vi "Launch Worker Loop.vi"(8 "error in (no error)":errorcluster, 11 "ErrorFormat":refnum<class "IErrorFormat.lvclass">) -> (0 "error out":errorcluster, 3 "Queue Reference":refnum<data-value>)   [LabVIEW 2018, in "MVA Framework.lvlib" / "Composed Log.lvlib" / "Application Logger.lvclass"]
uses:
  Application Logger.lvclass
  Worker Loop.vi
  Types/MessageCluster.ctl
  Composed Log.lvlib
  IErrorFormat/IErrorFormat.lvclass
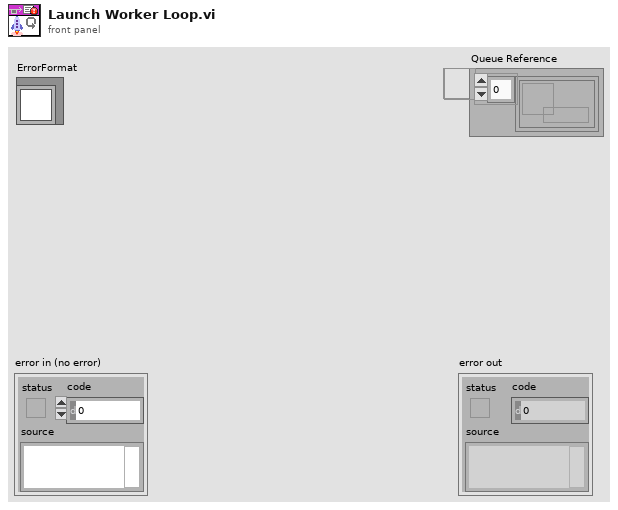
[diagram p1: front panel]
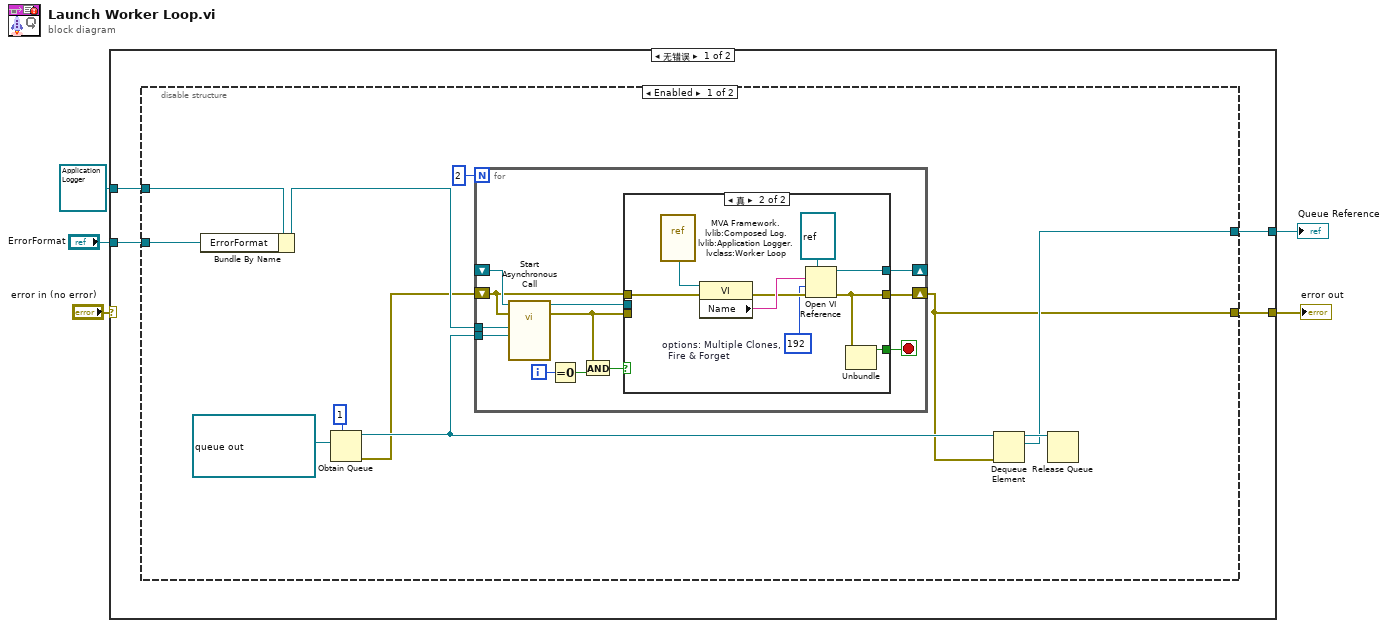
[diagram p0: block diagram]
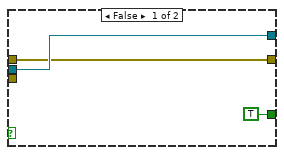
[diagram p2: hidden frame]
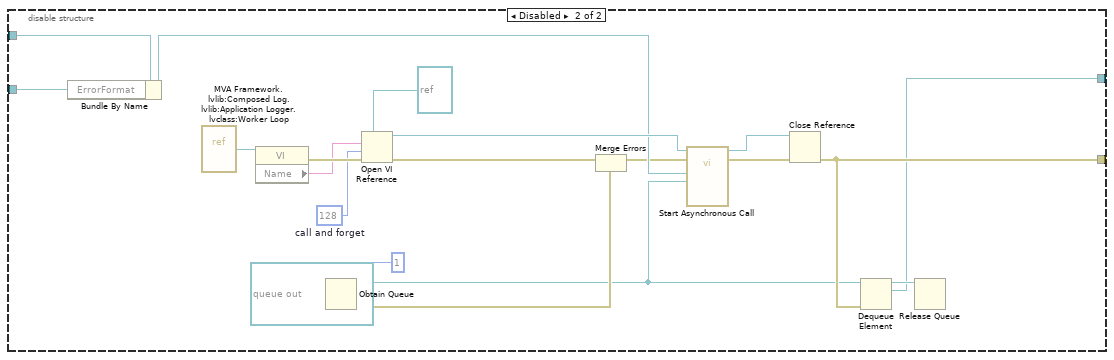
[diagram p3: hidden frame]
diagram:
  n1 = case shown="无错误" "error in (no error)" {
    selector: "error in (no error)" -> [_ w65]
    tunnel: [w8 w65] -> w4
    tunnel: refnum<class "Application Logger.lvclass"> refnum ("Application Logger In") -> [w9 _]
    tunnel: [w7 _] -> w1
    tunnel: "ErrorFormat" -> [w6 _]
    frame No Error {
      n2 = disable-structure shown="Enabled" {
        disable-tunnel: w9 -> [w20 w55]
        disable-tunnel: [w10 w54] -> w8
        disable-tunnel: [w18 w52] -> w7
        disable-tunnel: w6 -> [w16 w50]
        frame Enabled {
          n3 = Bundle By Name(cluster=w20, "ErrorFormat"=w16) -> (w17:refnum<class "Application Logger.lvclass">)
          n4 = Obtain Queue(max queue size (-1, unlimited)=1, element data type=refnum<data-value> refnum ("data value reference")) -> (queue out=w13:refnum<queue>, error out=w11:errorcluster)  [unwired: 3 in, 1 out]
          n5 = for {
            N: 2 -> [_]
            tunnel: w17 -> [w32]
            tunnel: w13 -> [w31]
            shift-right: [w26] -> _
            shift-left: _ -> [w30]
            shift-right: [w24] -> w10
            shift-left: w11 -> [w22]
            i -> [w29]
            stop <- w21 stop-if-true
            n6 = call-by-ref "Start Asynchronous Call"(reference=w30, error in=w22, "Return Queue"=w31, "Application Log"=w32) -> (reference out=w27:refnum<vi>, error out=w23:errorcluster)  [unwired: 10 in]
            n7 = Equal To 0?(x=w29) -> (x = 0?=w28:bool)
            n8 = And(x=w23, y=w28) -> (x .and. y?=w25:bool)
            n9 = case shown="真" w25 {
              tunnel: w27 -> [w35 _]
              tunnel: [w34 w37] -> w24
              tunnel: [w35 w40] -> w26
              tunnel: w22 -> [w34 w38]
              tunnel: w23 -> [_ _]
              tunnel: [TRUE ("status") w36] -> w21
              frame False {
              }
              frame True {
                w39 = 192  # options: Multiple Clones,   Fire & Forget
                n10 = vi-ref "MVA Framework.lvlib:Composed Log.lvlib:Application Logger.lvclass:Worker Loop.vi"() -> (w42:refnum<vi>)
                n11 = property class="VI"(reference=w42, error in=w38) -> (error out=w43:errorcluster, "Name"=w44:string)  [unwired: 1 out]
                n12 = Open VI Reference(type specifier VI Refnum (for type only)=refnum<vi> refnum, vi path=w44, options=w39, error in (no error)=w43) -> (vi reference=w40:refnum<vi>, error out=w37:errorcluster)  [unwired: 2 in]
                n13 = Unbundle(w37) -> ("status"=w36:bool)  [unwired: 2 out]
              }
            }
          }
          n14 = Dequeue Element(queue=w13, error in (no error)=w10) -> (queue out=w19:refnum<queue>, element=w18:refnum<data-value>)  [unwired: 1 in, 2 out]
          n15 = Release Queue(queue=w19) -> ()  [unwired: 2 in, 3 out]
        }
        frame Disabled {
          w61 = 128  # call and forget
          n16 = Bundle By Name(cluster=w55, "ErrorFormat"=w50) -> (w51:refnum<class "Application Logger.lvclass">)
          n17 = vi-ref "MVA Framework.lvlib:Composed Log.lvlib:Application Logger.lvclass:Worker Loop.vi"() -> (w64:refnum<vi>)
          n18 = property class="VI"(reference=w64) -> (error out=w63:errorcluster, "Name"=w60:string)  [unwired: 1 in, 1 out]
          n19 = Obtain Queue(max queue size (-1, unlimited)=1, element data type=refnum<data-value> refnum ("data value reference")) -> (queue out=w45:refnum<queue>, error out=w47:errorcluster)  [unwired: 3 in, 1 out]
          n20 = Open VI Reference(type specifier VI Refnum (for type only)=refnum<vi> refnum, vi path=w60, options=w61, error in (no error)=w63) -> (vi reference=w58:refnum<vi>, error out=w59:errorcluster)  [unwired: 2 in]
          n21 = Merge Errors(w59, w47) -> (w48:errorcluster)
          n22 = call-by-ref "Start Asynchronous Call"(reference=w58, error in=w48, "Return Queue"=w45, "Application Log"=w51) -> (reference out=w56:refnum<vi>, error out=w57:errorcluster)  [unwired: 10 in]
          n23 = Close Reference(reference=w56, error in (no error)=w57) -> (error out=w54:errorcluster)
          n24 = Dequeue Element(queue=w45, error in (no error)=w54) -> (queue out=w53:refnum<queue>, element=w52:refnum<data-value>)  [unwired: 1 in, 2 out]
          n25 = Release Queue(queue=w53) -> ()  [unwired: 2 in, 3 out]
        }
      }
    }
    frame Error {
    }
  }
  "error out" <- w4
  "Queue Reference" <- w1
